vi "DQMHModuleNode_Create.vi"(0 "reference in":refnum<class "DQMHModuleNode.lvclass">, 5 "error in (no error)":errorcluster) -> (14 "reference out":refnum<class "DQMHModuleNode.lvclass">, 19 "error out":errorcluster)   [LabVIEW 2014, in "DQMHModuleNode.lvclass"]
doc: "Creates and initializes a new ClassNode object.\n\nThis object should be destroyed using a ClassNode destructor VI or a virtual base class destructor VI.\n\n[GOOP 2.1]"
uses:
  <resource>/Framework/Providers/Open_GDS/UML/DQMHModuleNode_class/DQMHModuleNode.lvclass
  <resource>/Framework/Providers/Open_GDS/UML/MultiLineString_class/SizeType.ctl
  <resource>/Framework/Providers/Open_GDS/UML/MultiLineString_class/JustificationType.ctl
  <resource>/Framework/Providers/Open_GDS/UML/General/Rectangle/Rectangle Rectangle2D.ctl
  <resource>/Framework/Providers/Open_GDS/UML/RectangularNode_class/RectangularNode.lvclass
  <resource>/Framework/Providers/Open_GDS/UML/MultiLineString_class/MultiLineString.lvclass
panel:
  # "The input reference should only\nbe wired when this method is called\nby a sub class constructor."
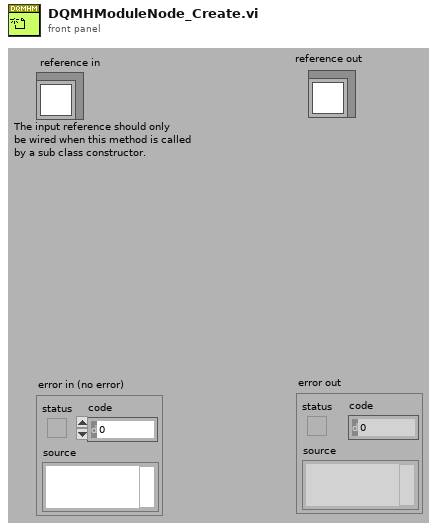
[diagram p1: front panel]
types:
  T1 = typedef "Rectangle Rectangle2D.ctl" = cluster{"x":dbl, "y":dbl, "width":dbl, "height":dbl}
  T2 = typedef "MultiLineString.lvclass/SizeType.ctl" = enum16{"LARGE", "NORMAL", "SMALL"}
  T3 = typedef "MultiLineString.lvclass/JustificationType.ctl" = enum16{"LEFT", "CENTER", "RIGHT"}
  T4 = typedef "DQMHModuleNode.lvclass/ObjectAttributes.ctl" = cluster{"DescriptionHeight":dbl, "InternalDataHeight":dbl, "EventsHeight":dbl, "Name":refnum<class "MultiLineString.lvclass">, "Description":refnum<class "MultiLineString.lvclass">, "InternalData":refnum<class "MultiLineString.lvclass">, "Events":refnum<class "MultiLineString.lvclass">, "showDescription":bool, "showInternalData":bool, "showEvents":bool, "DEFAULT_ROUNDING":i32, "DEFAULT_WIDTH":i32, "DEFAULT_HEIGHT":i32, "ClassPath":path, "Template":string, "Icon":u8[][]}
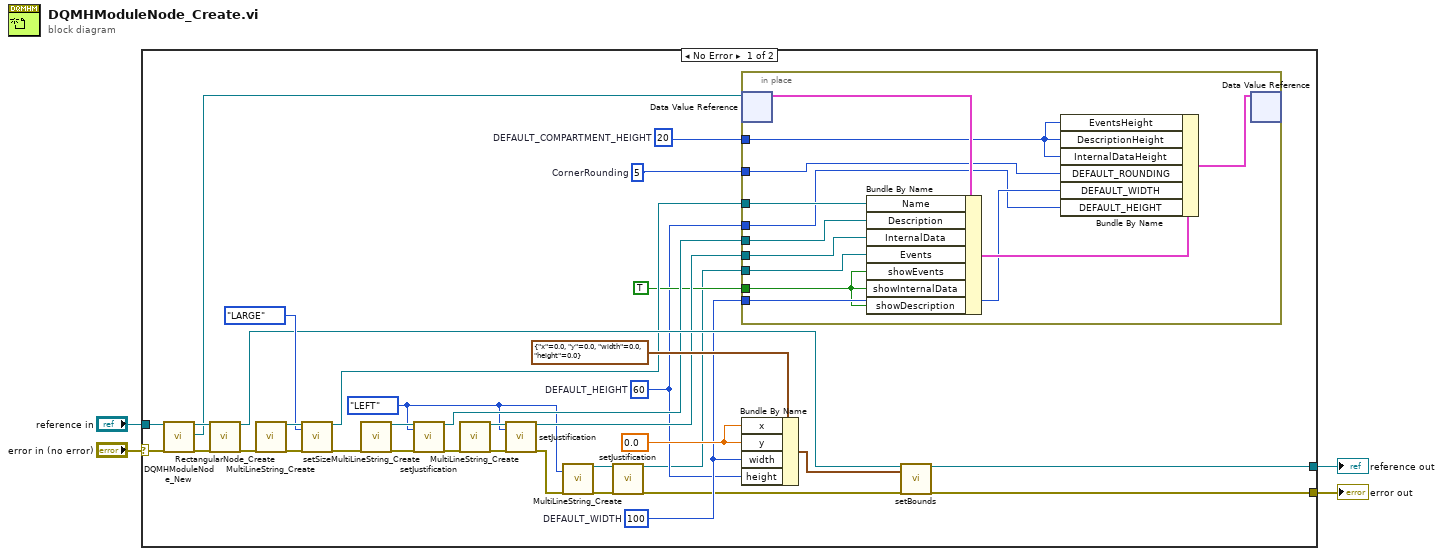
[diagram p0: block diagram]
diagram:
  n1 = case shown="No Error" "error in (no error)" {
    selector: "error in (no error)" -> [w39 w53]
    tunnel: [w13 w52] -> w4
    tunnel: [w12 w53] -> w3
    tunnel: "reference in" -> [w38 w52]
    frame No Error {
      w5 = 5  # CornerRounding
      w22 = 0.0 ("x")
      w7 = JustificationType."LEFT" ("justification")
      w15 = 60  # DEFAULT_HEIGHT
      w16 = 100  # DEFAULT_WIDTH
      w17 = 20  # DEFAULT_COMPARTMENT_HEIGHT
      n2 = call <resource>:"DQMHModuleNode_New.vi"("reference in"=w38, "error in (no error)"=w39) -> ("reference out"=w36:refnum<class "DQMHModuleNode.lvclass">, "DVRRefOut"=w14:refnum<data-value>, "error out"=w37:errorcluster)  [unwired: 2 in, 13 out]
      n3 = call <resource>:"RectangularNode_Create.vi"("reference"=w36, "error in (no error)"=w37) -> ("reference out"=w25:refnum<class "DQMHModuleNode.lvclass">, "error out"=w35:errorcluster)  [unwired: 1 in, 15 out]
      n4 = call <resource>:"MultiLineString_Create.vi"("error in (no error)"=w35) -> ("reference out"=w30:refnum<class "MultiLineString.lvclass">, "error out"=w29:errorcluster)  [unwired: 2 in, 15 out]
      n5 = call <resource>:"setSize.vi"("reference"=w30, "size"=SizeType."LARGE", "error in (no error)"=w29) -> ("reference out"=w21:refnum<class "MultiLineString.lvclass">, "error out"=w28:errorcluster)  [unwired: 15 out]
      n6 = call <resource>:"MultiLineString_Create.vi"("error in (no error)"=w28) -> ("reference out"=w34:refnum<class "MultiLineString.lvclass">, "error out"=w33:errorcluster)  [unwired: 2 in, 15 out]
      n7 = call <resource>:"setJustification.vi"("reference"=w34, "justification"=w7, "error in (no error)"=w33) -> ("reference out"=w20:refnum<class "MultiLineString.lvclass">, "error out"=w27:errorcluster)  [unwired: 15 out]
      n8 = call <resource>:"MultiLineString_Create.vi"("error in (no error)"=w27) -> ("reference out"=w32:refnum<class "MultiLineString.lvclass">, "error out"=w31:errorcluster)  [unwired: 2 in, 15 out]
      n9 = call <resource>:"setJustification.vi"("reference"=w32, "justification"=w7, "error in (no error)"=w31) -> ("reference out"=w19:refnum<class "MultiLineString.lvclass">, "error out"=w11:errorcluster)  [unwired: 15 out]
      n10 = call <resource>:"MultiLineString_Create.vi"("GAP"=w7, "error in (no error)"=w11) -> ("reference out"=w8:refnum<class "MultiLineString.lvclass">, "error out"=w10:errorcluster)  [unwired: 1 in, 15 out]
      n11 = call <resource>:"setJustification.vi"("reference"=w8, "error in (no error)"=w10) -> ("reference out"=w6:refnum<class "MultiLineString.lvclass">, "error out"=w9:errorcluster)  [unwired: 1 in, 15 out]
      n12 = in-place {
        in-place-border: w21 -> [w50]
        in-place-border: w20 -> [w49]
        in-place-border: w19 -> [w48]
        in-place-border: TRUE ("showMethods") -> [w41]
        in-place-border: w17 -> [w40]
        in-place-border: w5 -> [w46]
        in-place-border: w16 -> [w45]
        in-place-border: w15 -> [w44]
        in-place-border: w6 -> [w42]
        n13 = in-place-dvr #1(w14) -> (w51:T4)  [unwired: 1 out]
        n14 = Bundle By Name(cluster=w51, "Name"=w50, "Description"=w49, "InternalData"=w48, "Events"=w42, "showEvents"=w41, "showInternalData"=w41, "showDescription"=w41) -> (w47:T4)
        n15 = Bundle By Name(cluster=w47, "EventsHeight"=w40, "DescriptionHeight"=w40, "InternalDataHeight"=w40, "DEFAULT_ROUNDING"=w46, "DEFAULT_WIDTH"=w45, "DEFAULT_HEIGHT"=w44) -> (w43:T4)
        n16 = in-place-dvr #1(w43) -> ()  [unwired: 2 out]
      }
      n17 = Bundle By Name(cluster=T1 {"x"=0.0, "y"=0.0, "width"=0.0, "height"=0.0} ("bounds"), "x"=w22, "y"=w22, "width"=w16, "height"=w15) -> (w24:T1)
      n18 = call-dynamic "setBounds.vi"("reference"=w25, "bounds"=w24, "error in (no error)"=w9) -> ("reference out"=w13:refnum<class "DQMHModuleNode.lvclass">, "error out"=w12:errorcluster)  [unwired: 15 in]
    }
    frame Error {
    }
  }
  "error out" <- w3
  "reference out" <- w4
